vi "GetSubSettingPath.vi"(10 "settings file name":string, 11 "LabVIEW Data Path":path) -> (0 "folder":string, 3 "settings file path":path)   [LabVIEW 2022 SP3]
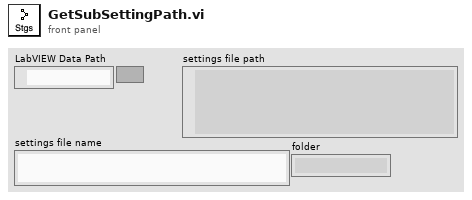
[diagram p1: front panel]
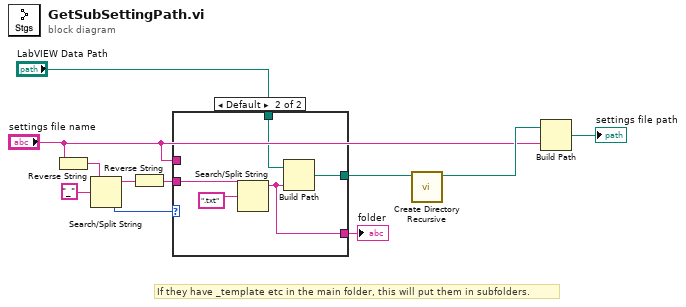
[diagram p0: block diagram]
diagram:
  # "If they have _template etc in the main folder, this will put them in subfolders."
  n1 = Reverse String(1:"settings file name") -> (0:w6:string)
  n2 = Search/Split String(string=w6, search string/char (-)="_" ("y")) -> (substring before match=w8:string, offset of match=w7:i32)  [unwired: 1 in, 1 out]
  n3 = Reverse String(1:w8) -> (0:w9:string)
  n4 = case shown="Default" w7 {
    tunnel: w9 -> [_ w18]
    tunnel: "LabVIEW Data Path" -> [w13 w16]
    tunnel: [w13 w15] -> w10
    tunnel: [w12 w14] -> w2
    tunnel: "settings file name" -> [w12 _]
    frame -1 {
    }
    frame Default {
      n5 = Search/Split String(string=w18, search string/char (-)=".txt" ("y")) -> (substring before match=w14:string)  [unwired: 1 in, 2 out]
      n6 = Build Path(base path=w16, name or relative path=w14) -> (appended path=w15:path)
    }
  }
  "folder" <- w2
  n7 = call <vilib>:"Create Directory Recursive.vi"("directory"=w10) -> ("directory copy"=w11:path)  [unwired: 4 in, 2 out]
  n8 = Build Path(base path=w11, name or relative path="settings file name") -> (appended path=→"settings file path":path)
